vi "Halvorsen_2D_All.vi"(11 "Initial Conditions":ext[](array[numeric])=[0.1, 0.0, 0.1]) -> ()   [LabVIEW 2016]
panel:
  in  "Tab Control":T1(tab)=enum."Time Domain"
  out "Exponent Behavior":cluster{ext, dbl}(graph)={0.0040208082977662581687, 0.0}
  out "Time Domain":ext[][](graph)
  out "Difference":ext[][](graph)
  out "Lyapunov":ext[][](graph)
  in  "Initial Conditions Inc":ext[](array[numeric])=[1e-10, 1e-10, 1e-10]
  out "Histogram":dbl[][](graph)=[[23.0, 22.0, 11.0, 12.0, 15.0, 1.0, 1.0, 13.0, 5.0, 1.0, 5.0, 4.0, 3.0, 4.0, 1.0, 3.0, 1.0], [20.0, 12.0, 13.0, 10.0, 6.0, 8.0, 12.0, 13.0, 9.0, 4.0, 6.0, 8.0, 1.0, 1.0, 1.0, 1.0, 1.0], [19.0, 17.0, 14.0, 7.0, 12.0, 14.0, 14.0, 12.0, 1.0, 6.0, 10.0, 1.0, 3.0, 1.0, 1.0, 1.0, 1.0], [18.0, 11.0, 16.0, 14.0, 10.0, 11.0, 11.0, 10.0, 4.0, 9.0, 2.0, 7.0, 3.0, 1.0, 1.0, 1.0, 1.0], [15.0, 21.0, 11.0, 16.0, 12.0, 11.0, 7.0, 13.0, 8.0, 3.0, 6.0, 5.0, 2.0, 1.0, 1.0, 1.0, 1.0], [21.0, 13.0, 15.0, 9.0, 13.0, 2.0, 5.0, 11.0, 14.0, 10.0, 10.0, 1.0, 1.0, 1.0, 1.0, 1.0, 1.0], [15.0, 18.0, 15.0, 14.0, 13.0, 2.0, 9.0, 11.0, 6.0, 4.0, 4.0, 1.0, 1.0, 1.0, 6.0, 1.0, 1.0], [17.0, 17.0, 18.0, 16.0, 17.0, 1.0, 2.0, 4.0, 4.0, 5.0, 5.0, 1.0, 7.0, 7.0, 2.0, 2.0, 1.0], [18.0, 8.0, 16.0, 10.0, 12.0, 1.0, 15.0, 2.0, 3.0, 4.0, 1.0, 8.0, 7.0, 2.0, 3.0, 1.0, 1.0], [20.0, 15.0, 13.0, 14.0, 6.0, 10.0, 9.0, 9.0, 6.0, 4.0, 3.0, 12.0, 2.0, 2.0, 2.0, 5.0, 1.0], [22.0, 8.0, 14.0, 2.0, 9.0, 8.0, 7.0, 9.0, 6.0, 3.0, 3.0, 6.0, 8.0, 10.0, 2.0, 1.0, 1.0], [21.0, 3.0, 14.0, 12.0, 7.0, 11.0, 15.0, 14.0, 14.0, 3.0, 3.0, 3.0, 2.0, 2.0, 2.0, 2.0, 2.0], [20.0, 12.0, 2.0, 3.0, 2.0, 4.0, 13.0, 10.0, 3.0, 3.0, 4.0, 2.0, 2.0, 2.0, 2.0, 2.0, 2.0], [22.0, 12.0, 2.0, 4.0, 3.0, 13.0, 3.0, 3.0, 3.0, 2.0, 2.0, 2.0, 2.0, 2.0, 2.0, 2.0, 2.0], [15.0, 7.0, 3.0, 4.0, 3.0, 2.0, 2.0, 2.0, 2.0, 2.0, 2.0, 2.0, 2.0, 2.0, 2.0, 2.0, 2.0], [20.0, 2.0, 3.0, 3.0, 3.0, 2.0, 2.0, 2.0, 2.0, 2.0, 2.0, 2.0, 2.0, 2.0, 2.0, 2.0, 2.0], [17.0, 2.0, 3.0, 3.0, 3.0, 2.0, 2.0, 2.0, 2.0, 2.0, 2.0, 2.0, 2.0, 2.0, 2.0, 2.0, 2.0]]
  out "KDE":dbl[][](graph)=[[24.0, 23.0, 12.0, 13.0, 15.0, 2.0, 2.0, 13.0, 4.0, 2.0, 6.0, 5.0, 4.0, 5.0, 2.0, 4.0, 2.0], [21.0, 12.0, 14.0, 11.0, 7.0, 8.0, 13.0, 14.0, 9.0, 4.0, 7.0, 9.0, 1.0, 1.0, 1.0, 1.0, 1.0], [18.0, 18.0, 15.0, 8.0, 13.0, 14.0, 15.0, 11.0, 2.0, 7.0, 11.0, 2.0, 4.0, 1.0, 1.0, 1.0, 1.0], [17.0, 12.0, 17.0, 14.0, 11.0, 12.0, 12.0, 9.0, 2.0, 10.0, 2.0, 7.0, 2.0, 1.0, 1.0, 1.0, 1.0], [15.0, 20.0, 12.0, 12.0, 13.0, 12.0, 8.0, 13.0, 3.0, 4.0, 7.0, 6.0, 1.0, 1.0, 1.0, 1.0, 1.0], [22.0, 14.0, 16.0, 7.0, 13.0, 1.0, 5.0, 12.0, 13.0, 7.0, 9.0, 1.0, 1.0, 1.0, 1.0, 1.0, 1.0], [15.0, 18.0, 15.0, 14.0, 14.0, 2.0, 9.0, 8.0, 6.0, 3.0, 4.0, 1.0, 1.0, 1.0, 7.0, 1.0, 1.0], [16.0, 16.0, 17.0, 16.0, 17.0, 1.0, 2.0, 3.0, 3.0, 3.0, 3.0, 1.0, 8.0, 8.0, 2.0, 2.0, 1.0], [17.0, 6.0, 16.0, 11.0, 11.0, 1.0, 15.0, 2.0, 3.0, 3.0, 1.0, 7.0, 8.0, 2.0, 3.0, 1.0, 1.0], [14.0, 15.0, 9.0, 13.0, 4.0, 6.0, 6.0, 8.0, 6.0, 3.0, 3.0, 13.0, 2.0, 2.0, 2.0, 4.0, 1.0], [21.0, 9.0, 13.0, 2.0, 8.0, 5.0, 6.0, 4.0, 5.0, 3.0, 3.0, 4.0, 7.0, 8.0, 2.0, 1.0, 1.0], [21.0, 3.0, 14.0, 10.0, 3.0, 7.0, 13.0, 13.0, 13.0, 3.0, 3.0, 3.0, 2.0, 2.0, 2.0, 2.0, 2.0], [20.0, 11.0, 2.0, 3.0, 2.0, 3.0, 10.0, 10.0, 3.0, 3.0, 4.0, 2.0, 2.0, 2.0, 2.0, 2.0, 2.0], [19.0, 12.0, 2.0, 3.0, 3.0, 11.0, 3.0, 3.0, 3.0, 2.0, 2.0, 2.0, 2.0, 2.0, 2.0, 2.0, 2.0], [12.0, 6.0, 3.0, 3.0, 3.0, 3.0, 2.0, 2.0, 2.0, 2.0, 2.0, 2.0, 2.0, 2.0, 2.0, 2.0, 2.0], [19.0, 3.0, 3.0, 3.0, 3.0, 2.0, 2.0, 2.0, 2.0, 2.0, 2.0, 2.0, 2.0, 2.0, 2.0, 2.0, 2.0], [15.0, 2.0, 3.0, 3.0, 3.0, 2.0, 2.0, 2.0, 2.0, 2.0, 2.0, 2.0, 2.0, 2.0, 2.0, 2.0, 2.0]]
  in  "X_Inc":dbl[](array[numeric])=[0.02, 0.0, 0.0]
  in  "Final_X":dbl=0.35
  in  "Param_X":i32
  in  "Param_Y":i32=1
  in  "Final Y":dbl=0.35
  in  "Y_Inc":dbl[](array[numeric])=[0.0, 0.02, 0.0]
  in  "Parameter_Vector":ext[](array[numeric])=[0.01, 0.01, 0.1]
  out "Current_Param":ext[](array[numeric])=[0.01, 0.29000000000000000582, 0.1]
  in  "Variable":u16(ring) items=["x", "y", "z"]
  in  "Время, с":ext=300.0
  in  "Hmin":ext=0.00099999999999999999996
  in  "Hmax":ext=1.0
  in  "tolerance":ext=1e-12
  in  "Шаг h, с":ext=0.01
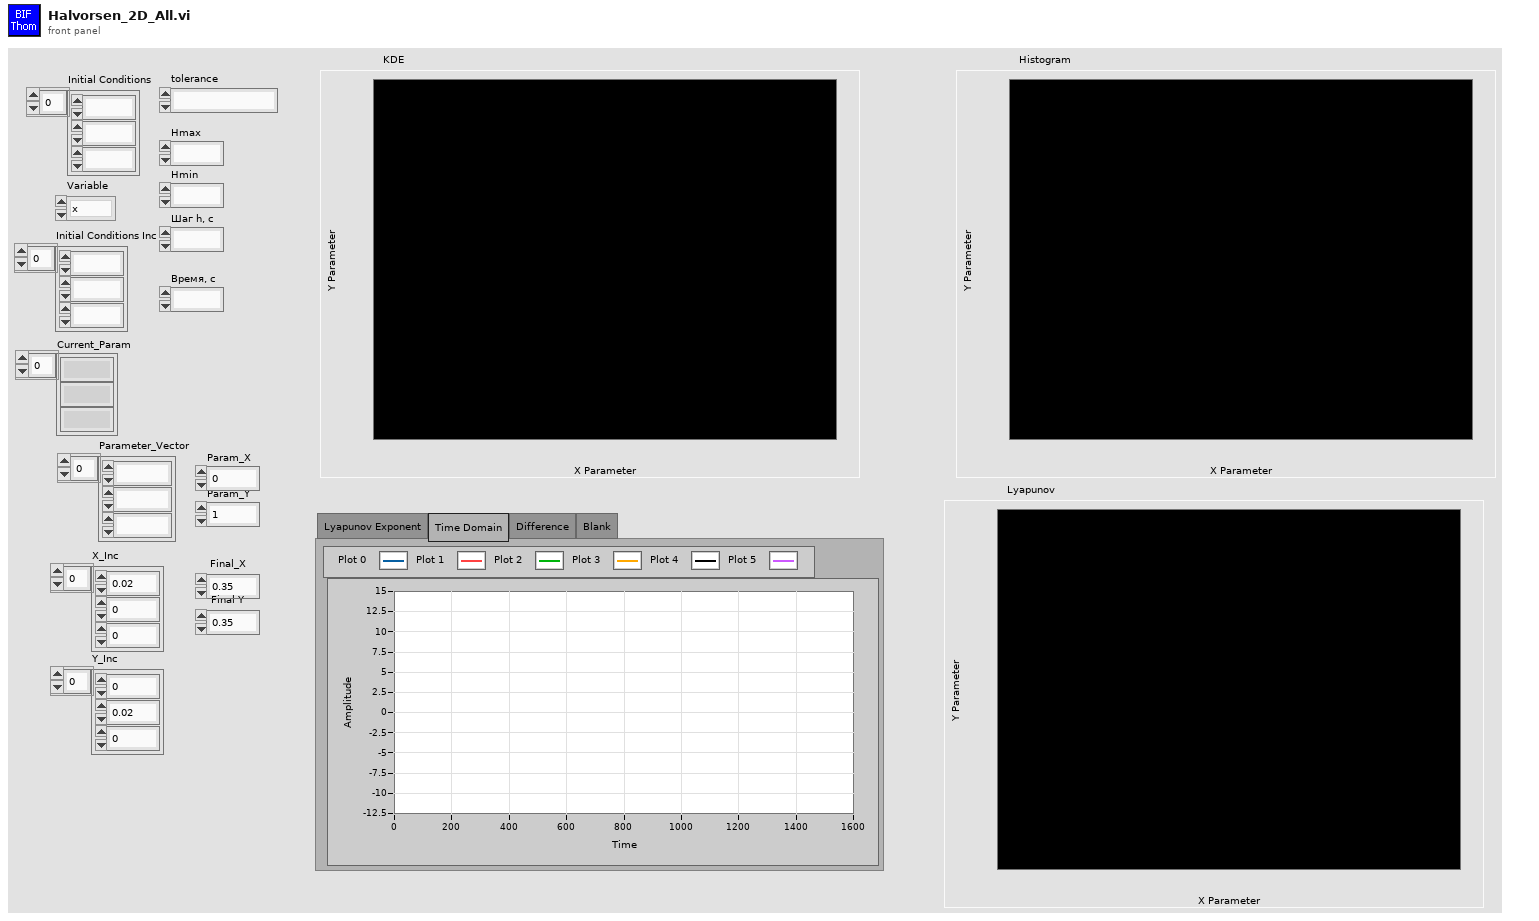
[diagram p1: front panel]
types:
  T1 = enum32{"Lyapunov Exponent", "Time Domain", "Difference", "Blank"}
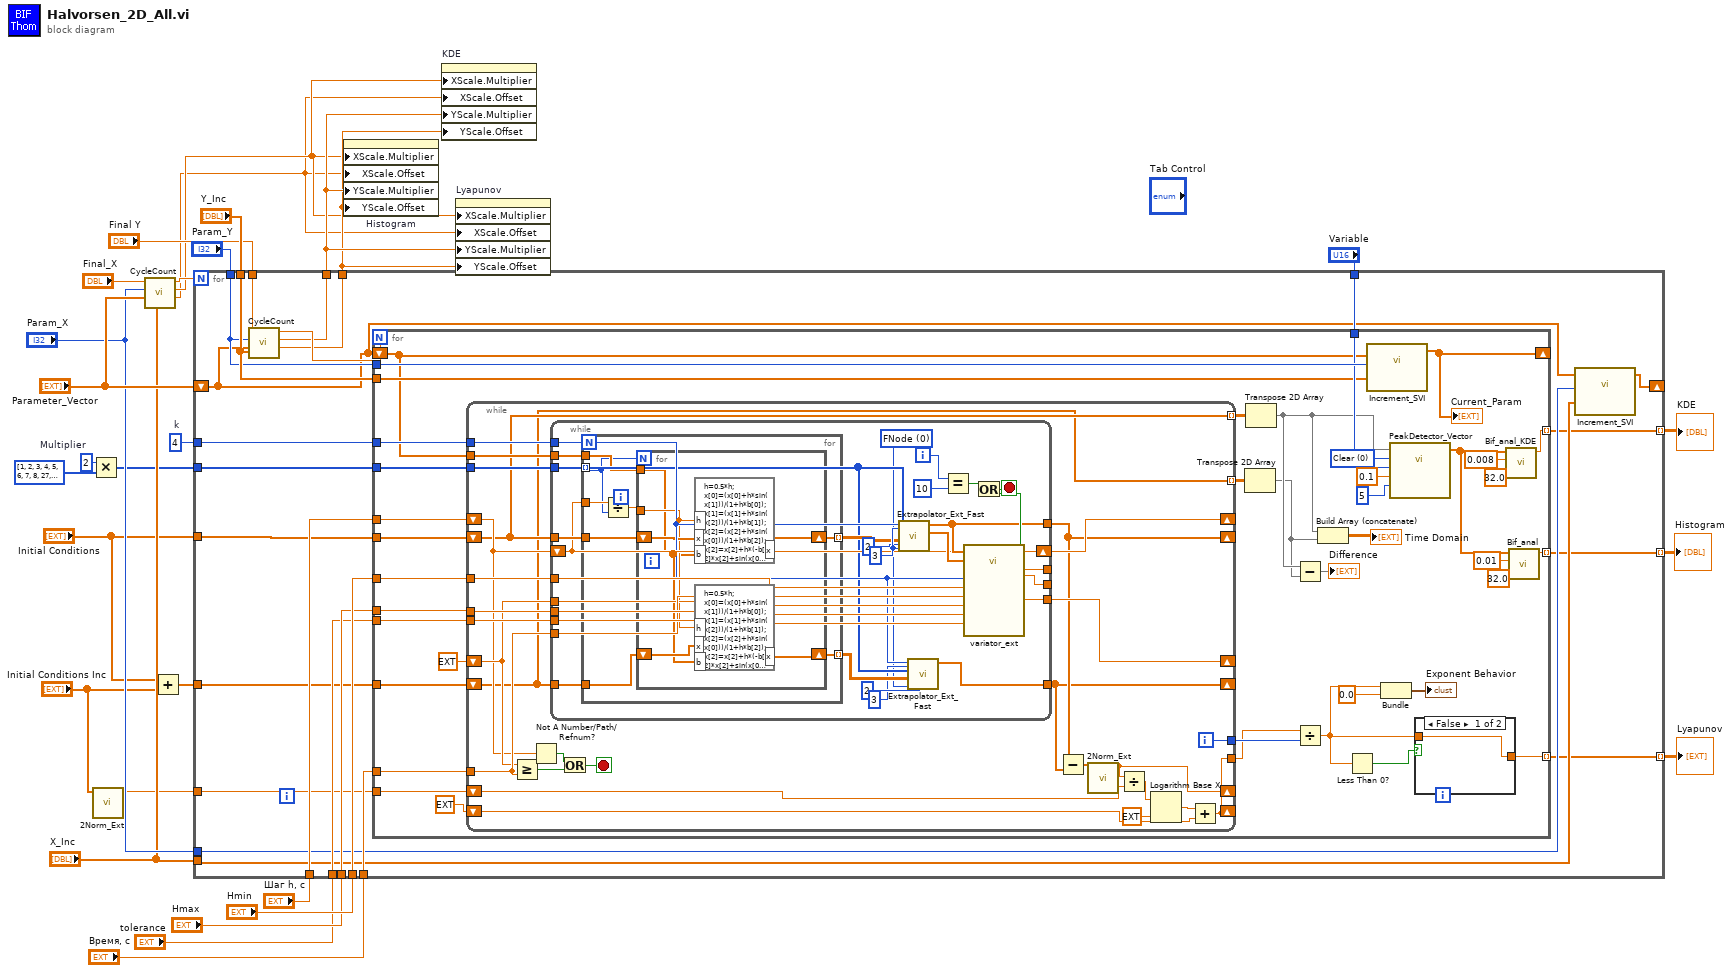
[diagram p0: block diagram]
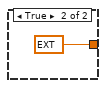
[diagram p2: hidden frame]
diagram:
  w6 = 4  # k
  w14 = 2  # Multiplier
  n1 = Multiply(x=w14, y=i32[] [1, 2, 3, 4, 5, 6, 7, 8, 27, 30, 33] ("n")) -> (x*y=w12:i32[])
  n2 = call "2Norm_Ext.vi"("Input vector"="Initial Conditions Inc") -> ("2 Norm"=w9:ext)  [unwired: 10 in]
  n3 = call "CycleCount.vi"("Increment_Vector"="X_Inc", "Parameter_Vector"="Parameter_Vector", "Parameter Number"="Param_X", "Final_Parameter_Value"="Final_X") -> ("Parameter Offset"=w1:ext, "Parameter Multiplier"=w2:dbl, "Cycle Count"=w24:ext)  [unwired: 5 in]
  n4 = Add(x="Initial Conditions", y="Initial Conditions Inc") -> (x+y=w10:ext[])
  n5 = for {
    N: w24 -> [_]
    tunnel: "Шаг h, с" -> [w53]
    tunnel: "Initial Conditions" -> [w52]
    tunnel: "Hmin" -> [w51]
    tunnel: "Hmax" -> [w50]
    tunnel: "tolerance" -> [w49]
    tunnel: "Время, с" -> [w48]
    shift-right: [w34] -> _
    shift-left: "Parameter_Vector" -> [w30]
    tunnel: "Param_X" -> [w47]
    tunnel: "X_Inc" -> [w46]
    tunnel: [w45] -> w19 mode=indexing
    tunnel: "Final Y" -> [w44]
    tunnel: "Param_Y" -> [w41]
    tunnel: "Y_Inc" -> [w42]
    tunnel: "Variable" -> [w40]
    tunnel: w12 -> [w39]
    tunnel: [w38] -> w11 mode=indexing
    tunnel: w10 -> [w37]
    tunnel: [w36] -> w5 mode=indexing
    tunnel: w9 -> [w35]
    tunnel: w6 -> [w33]
    tunnel: [w32] -> w4
    tunnel: [w31] -> w3
    n6 = call "CycleCount.vi"("Increment_Vector"=w42, "Parameter_Vector"=w30, "Parameter Number"=w41, "Final_Parameter_Value"=w44) -> ("Parameter Offset"=w31:ext, "Parameter Multiplier"=w32:dbl, "Cycle Count"=w43:ext)  [unwired: 5 in]
    n7 = for {
      N: w43 -> [_]
      tunnel: w33 -> [w74]
      tunnel: w53 -> [w72]
      tunnel: w48 -> [w71]
      tunnel: w49 -> [w69]
      tunnel: w51 -> [w73]
      tunnel: w50 -> [w70]
      tunnel: w39 -> [w75]
      tunnel: w52 -> [w77]
      shift-right: [w87] -> _
      shift-left: w30 -> [w54]
      tunnel: w41 -> [w90]
      tunnel: w42 -> [w67]
      tunnel: [w89] -> w45 mode=indexing
      tunnel: w40 -> [w88]
      tunnel: [w81] -> w38 mode=indexing
      tunnel: w37 -> [w76]
      tunnel: [w62] -> w36 mode=indexing
      tunnel: w35 -> [w68]
      w93 = u16 0 items=["Clear", "Absolute", "Positive"] ("Signal Mode")
      n8 = while {
        shift-right: [w100] -> _
        shift-left: w77 -> [w106]
        tunnel: w75 -> [w120]
        tunnel: w74 -> [w119]
        shift-right: [w115] -> _
        shift-left: w72 -> [w108]
        shift-right: [w112] -> _
        shift-left: ext 0.0 ("New time") -> [w113]
        tunnel: w71 -> [w114]
        tunnel: w69 -> [w116]
        tunnel: w73 -> [w118]
        tunnel: w70 -> [w117]
        tunnel: w54 -> [w111]
        tunnel: [w106] -> w78 mode=indexing
        shift-right: [w99] -> _
        shift-left: w76 -> [w94]
        shift-right: [w97] -> _
        shift-left: w68 -> [w101]
        shift-right: [w96] -> _
        shift-left: ext 0.0 -> [w102]
        tunnel: [w96] -> w65
        tunnel: [w95] -> w66
        tunnel: [w94] -> w64 mode=indexing
        i -> [w95]
        stop <- w110 stop-if-true
        n9 = Greater Or Equal?(x=w113, y=w114) -> (x >= y?=w109:bool)
        n10 = Not A Number/Path/Refnum?(number/path/refnum=w108) -> (NaN/Path/Refnum?=w107:bool)
        n11 = while {
          tunnel: w118 -> [w144]
          tunnel: w117 -> [w147]
          tunnel: w116 -> [w143]
          tunnel: w119 -> [w127]
          tunnel: w120 -> [w126]
          tunnel: w106 -> [w145]
          shift-right: [w138] -> w115
          shift-left: w108 -> [w130]
          tunnel: [w130] -> _
          tunnel: [w137] -> _
          tunnel: [w136] -> w100
          tunnel: w114 -> [w135]
          tunnel: w113 -> [w134]
          tunnel: [w132] -> w112
          tunnel: w111 -> [w131]
          tunnel: w94 -> [w128]
          tunnel: [w122] -> w99
          i -> [w133]
          stop <- w139 stop-if-true
          w121 = u16 0 items=["FNode", "MathScript", "ECD8 Arrays", "ECD8 Fnode", "ECD8 FnodeDiv"] ("Ext.Type")
          n12 = for {
            N: w127 -> [_]
            tunnel: w126 -> [w152] mode=indexing
            tunnel: w130 -> [w157]
            tunnel: w145 -> [w155]
            tunnel: [w156] -> w146 mode=indexing
            tunnel: w131 -> [w153]
            tunnel: w128 -> [w151]
            tunnel: [w150] -> w125 mode=indexing
            n13 = Divide(x=w157, y=w152) -> (x/y=w154:ext)
            n14 = for {
              N: w152 -> [_]
              shift-right: [w163] -> w156
              shift-left: w155 -> [w162]
              tunnel: w154 -> [w160]
              tunnel: w153 -> [w158]
              shift-right: [w161] -> w150
              shift-left: w151 -> [w159]
              n15 = formula code="h=0.5*h;\nx[0]=(x[0]+h*sin(x[1]))/(1+h*b[0]);\nx[1]=(x[1]+h*sin(x[2]))/(1+h*b[1]);\nx[2]=(x[2]+h*sin(x[0]))/(1+h*b[2]);\nx[2]=x[2]+h*(-b[2]*x[2]+sin(x[0]));\nx[1]=x[1]+h*(-b[1]*x[1]+sin(x[2]));\nx[0]=x[0]+h*(-b[0]*x[0]+sin(x[1]));"("x"=w162, "b"=w158, "h"=w160) -> ("x"=w163:ext[])
              n16 = formula code="h=0.5*h;\nx[0]=(x[0]+h*sin(x[1]))/(1+h*b[0]);\nx[1]=(x[1]+h*sin(x[2]))/(1+h*b[1]);\nx[2]=(x[2]+h*sin(x[0]))/(1+h*b[2]);\nx[2]=x[2]+h*(-b[2]*x[2]+sin(x[0]));\nx[1]=x[1]+h*(-b[1]*x[1]+sin(x[2]));\nx[0]=x[0]+h*(-b[0]*x[0]+sin(x[1]));"("x"=w159, "b"=w158, "h"=w160) -> ("x"=w161:ext[])
            }
          }
          n17 = call "Extrapolator_Ext_Fast.vi"("Порядок экстраполятора"=2 ("Ext. Order"), "Dimension"=3 ("input variable"), "Ext.Type"=w121, "Х - нач. условия"=w146, "n"=w126, "k"=w127) -> ("TPrev"=w148:ext[], "Tout"=w136:ext[])  [unwired: 4 in]
          n18 = call "Extrapolator_Ext_Fast.vi"("Порядок экстраполятора"=2 ("Ext. Order"), "Dimension"=3 ("input variable"), "Ext.Type"=w121, "Х - нач. условия"=w125, "n"=w126, "k"=w127) -> ("Tout"=w122:ext[])  [unwired: 4 in, 1 out]
          n19 = Equal?(x=w133, y=10) -> (x = y?=w141:bool)
          n20 = call "variator_ext.vi"("Tout"=w136, "tolerance"=w143, "Hmax"=w147, "TPrev"=w148, "Шаг h, с"=w130, "Current time"=w134, "k"=w127, "Hmin"=w144, "tmax"=w135) -> ("Hnew"=w138:ext, "error estimation"=w137:ext, "New time"=w132:ext, "stop"=w140:bool)  [unwired: 3 in]
          n21 = Or(x=w141, y=w140) -> (x .or. y?=w139:bool)
        }
        n22 = Or(x=w107, y=w109) -> (x .or. y?=w110:bool)
        n23 = Subtract(x=w100, y=w99) -> (x-y=w98:ext[])
        n24 = call "2Norm_Ext.vi"("Input vector"=w98) -> ("2 Norm"=w97:ext)  [unwired: 10 in]
        n25 = Divide(x=w97, y=w101) -> (x/y=w105:ext)
        n26 = Logarithm Base X(1:ext 10.0 ("x"), 2:w105) -> (0:w104:ext)
        n27 = Add(x=w104, y=w102) -> (x+y=w96:ext)
      }
      n28 = Transpose 2D Array(2D array=w64) -> (transposed array=w56:ext[][])
      n29 = Transpose 2D Array(2D array=w78) -> (transposed array=w57:ext[][])
      n30 = Subtract(x=w57, y=w56) -> (x-y=→"Difference":ext[][])
      n31 = Divide(x=w65, y=w66) -> (x/y=w59:ext)
      n32 = Build Array (concatenate)(w57, w56) -> (→"Time Domain":ext[][])
      n33 = Less Than 0?(x=w59) -> (x < 0?=w63:bool)
      n34 = call "Increment_SVI.vi"("Increment_Vector"=w67, "Param_Index"=w90, "Parameter_Vector"=w54) -> ("Parameters_Out"=w87:ext[])  [unwired: 7 in, 1 out]
      "Current_Param" <- w87
      n35 = Bundle(w59, 0.0) -> (→"Exponent Behavior":cluster{ext, dbl})  [unwired: 1 in]
      n36 = call "PeakDetector_Vector.vi"("threshold"=0.1, "FWD cut length"=5, "Variable_Num"=w88, "Signal Mode"=w93, "Input signal"=w57) -> ("Out signal"=w86:dbl[])  [unwired: 5 in, 1 out]
      n37 = case shown="False" w63 {
        tunnel: [w164 ext 1e-8] -> w62
        tunnel: w59 -> [w164 _]
        frame False {
        }
        frame True {
        }
      }
      n38 = call "Bif_anal_KDE.vi"("n"=32.0, "Manual h"=0.008 ("Treshold"), "X"=w86) -> ("Y"=w89:dbl)  [unwired: 7 in, 1 out]
      n39 = call "Bif_anal.vi"("n"=32.0, "Treshold"=0.01, "X"=w86) -> ("Y"=w81:dbl)  [unwired: 7 in, 1 out]
    }
    n40 = call "Increment_SVI.vi"("Increment_Vector"=w46, "Param_Index"=w47, "Parameter_Vector"=w30) -> ("Parameters_Out"=w34:ext[])  [unwired: 7 in, 1 out]
  }
  "KDE" <- w19
  "Histogram" <- w11
  "Lyapunov" <- w5
  n41 = property on="Histogram" class="IntGraph (strict)"("XScale.Multiplier"=w2, "XScale.Offset"=w1, "YScale.Multiplier"=w4, "YScale.Offset"=w3) -> ()  [unwired: 2 in, 2 out]
  n42 = property on="KDE" class="IntGraph (strict)"("XScale.Multiplier"=w2, "XScale.Offset"=w1, "YScale.Multiplier"=w4, "YScale.Offset"=w3) -> ()  [unwired: 2 in, 2 out]
  n43 = property on="Lyapunov" class="IntGraph (strict)"("XScale.Multiplier"=w2, "XScale.Offset"=w1, "YScale.Multiplier"=w4, "YScale.Offset"=w3) -> ()  [unwired: 2 in, 2 out]
